vi "SUB Json_to_cluster.vi"(5 "path":string[](array[string]), 11 "file path (dialog if empty)":path) -> (3 "Meta_FFR_AVG":T1)   [LabVIEW 2017]
uses:
  <vilib>/Utility/file.llb/Read Delimited Spreadsheet (string).vi
panel:
  in  "Data":T1
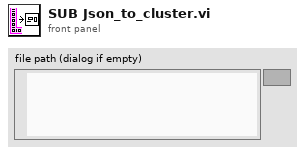
[diagram p1: front panel]
types:
  T1 = cluster{"MetaData":cluster{"Examen":string, "rejected":u16, "accepted":dbl, "time string":string, "date string":string, "ExportFolder":string, "RZ6_filter":cluster{"HP V":dbl, "HP H":dbl, "LP V":dbl, "LP H":dbl}, "RCX_path":string, "BERA":cluster{"DPOAE":dbl, "Threshold[dB]":dbl, "ClickABR":dbl, "Commentaire":string, "Seuils":u16}, "Stimulus":cluster{"F2":dbl, "F1":dbl, "Level[dB]":dbl, "V2[V]":dbl, "V1[V]":dbl, "L2[dB]":dbl, "L1[dB]":dbl, "Type":string}, "Patient":cluster{"Number":string, "Prenom":string, "Nom":string, "Oreille ":string, "Birthday":cluster{"Day":dbl, "Year":dbl, "Month":dbl}}}, "FFR":cluster{"Channel-V":cluster{"EFR":cluster{"Analysis":cluster{"S/N":string, "FFT":string, "Lenght":string, "Latency":string, "Frequency":string, "SC":string, "PLV":string, "InstAmpl":dbl[], "InstPhase":dbl[]}, "AVG":cluster{"Waveform":dbl[]}}, "EFR**":cluster{"Analysis":cluster{"S/N":string, "FFT":string, "Lenght":string, "Latency":string, "Frequency":string, "SC":string, "PLV":string, "InstAmpl":dbl[], "InstPhase":dbl[]}, "AVG":cluster{"Waveform":dbl[]}}, "EFR***":cluster{"Analysis":cluster{"S/N":string, "FFT":string, "Lenght":string, "Latency":string, "Frequency":string, "SC":string, "PLV":string, "InstAmpl":dbl[], "InstPhase":dbl[]}, "AVG":cluster{"Waveform":dbl[]}}, "F1":cluster{"Analysis":cluster{"S/N":string, "FFT":string, "Lenght":string, "Latency":string, "Frequency":string, "SC":string, "PLV":string, "InstAmpl":dbl[], "InstPhase":dbl[]}, "AVG":cluster{"Waveform":dbl[]}}, "F2":cluster{"Analysis":cluster{"S/N":string, "FFT":string, "Lenght":string, "Latency":string, "Frequency":string, "SC":string, "PLV":string, "InstAmpl":dbl[], "InstPhase":dbl[]}, "AVG":cluster{"Waveform":dbl[]}}, "CDT":cluster{"Analysis":cluster{"S/N":string, "FFT":string, "Lenght":string, "Latency":string, "Frequency":string, "SC":string, "PLV":string, "InstAmpl":dbl[], "InstPhase":dbl[]}, "AVG":cluster{"Waveform":dbl[]}}, "CDT*":cluster{"Analysis":cluster{"S/N":string, "FFT":string, "Lenght":string, "Latency":string, "Frequency":string, "SC":string, "PLV":string, "InstAmpl":dbl[], "InstPhase":dbl[]}, "AVG":cluster{"Waveform":dbl[]}}, "ABR":cluster{"Analysis":cluster{"S/N":string, "FFT":string, "Lenght":string, "Latency":string, "Frequency":string, "SC":string, "PLV":string, "InstAmpl":dbl[], "InstPhase":dbl[]}, "AVG":cluster{"Waveform":dbl[]}}, "Noise":cluster{"Analysis":cluster{"S/N":string, "FFT":string, "Lenght":string, "Latency":string, "Frequency":string, "SC":string, "PLV":string, "InstAmpl":dbl[], "InstPhase":dbl[]}, "AVG":cluster{"Waveform":dbl[]}}}, "Channel-H":cluster{"EFR":cluster{"Analysis":cluster{"S/N":string, "FFT":string, "Lenght":string, "Latency":string, "Frequency":string, "SC":string, "PLV":string, "InstAmpl":dbl[], "InstPhase":dbl[]}, "AVG":cluster{"Waveform":dbl[]}}, "EFR**":cluster{"Analysis":cluster{"S/N":string, "FFT":string, "Lenght":string, "Latency":string, "Frequency":string, "SC":string, "PLV":string, "InstAmpl":dbl[], "InstPhase":dbl[]}, "AVG":cluster{"Waveform":dbl[]}}, "EFR***":cluster{"Analysis":cluster{"S/N":string, "FFT":string, "Lenght":string, "Latency":string, "Frequency":string, "SC":string, "PLV":string, "InstAmpl":dbl[], "InstPhase":dbl[]}, "AVG":cluster{"Waveform":dbl[]}}, "F1":cluster{"Analysis":cluster{"S/N":string, "FFT":string, "Lenght":string, "Latency":string, "Frequency":string, "SC":string, "PLV":string, "InstAmpl":dbl[], "InstPhase":dbl[]}, "AVG":cluster{"Waveform":dbl[]}}, "F2":cluster{"Analysis":cluster{"S/N":string, "FFT":string, "Lenght":string, "Latency":string, "Frequency":string, "SC":string, "PLV":string, "InstAmpl":dbl[], "InstPhase":dbl[]}, "AVG":cluster{"Waveform":dbl[]}}, "CDT":cluster{"Analysis":cluster{"S/N":string, "FFT":string, "Lenght":string, "Latency":string, "Frequency":string, "SC":string, "PLV":string, "InstAmpl":dbl[], "InstPhase":dbl[]}, "AVG":cluster{"Waveform":dbl[]}}, "CDT*":cluster{"Analysis":cluster{"S/N":string, "FFT":string, "Lenght":string, "Latency":string, "Frequency":string, "SC":string, "PLV":string, "InstAmpl":dbl[], "InstPhase":dbl[]}, "AVG":cluster{"Waveform":dbl[]}}, "ABR":cluster{"Analysis":cluster{"S/N":string, "FFT":string, "Lenght":string, "Latency":string, "Frequency":string, "SC":string, "PLV":string, "InstAmpl":dbl[], "InstPhase":dbl[]}, "AVG":cluster{"Waveform":dbl[]}}, "Noise":cluster{"Analysis":cluster{"S/N":string, "FFT":string, "Lenght":string, "Latency":string, "Frequency":string, "SC":string, "PLV":string, "InstAmpl":dbl[], "InstPhase":dbl[]}, "AVG":cluster{"Waveform":dbl[]}}}}}
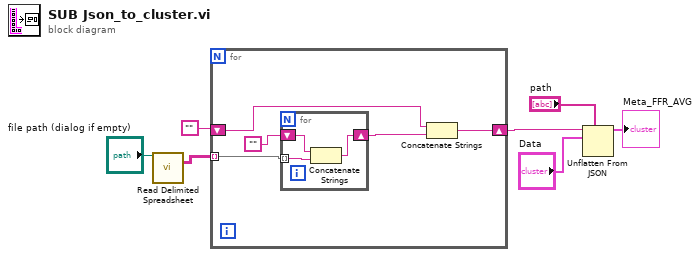
[diagram p0: block diagram]
diagram:
  n1 = call-poly <vilib>:"Read Delimited Spreadsheet.vi"("file path (dialog if empty)"="file path (dialog if empty)") -> ("all rows"=w7:string[][])  [unwired: 9 in, 5 out]
  n2 = for {
    tunnel: w7 -> [w12] mode=indexing
    shift-right: [w10] -> w5
    shift-left: "" -> [w9]
    n3 = for {
      tunnel: w12 -> [w13] mode=indexing
      shift-right: [w15] -> w11
      shift-left: "" -> [w14]
      n4 = Concatenate Strings(w14, w13) -> (w15:string)
    }
    n5 = Concatenate Strings(w9, w11) -> (w10:string)
  }
  n6 = Unflatten From JSON(path="path", JSON string=w5, type and defaults="Data") -> (value=→"Meta_FFR_AVG":T1)  [unwired: 4 in, 1 out]
